vi "Vision Compression AE.vi"(7 "Update":bool, 10 "Quality (750)":i32=750) -> (2 "Quality out":i32, 5 "Compression":i32)   [LabVIEW 2023]
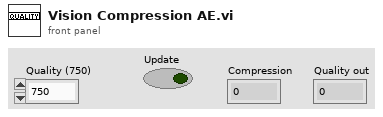
[diagram p1: front panel]
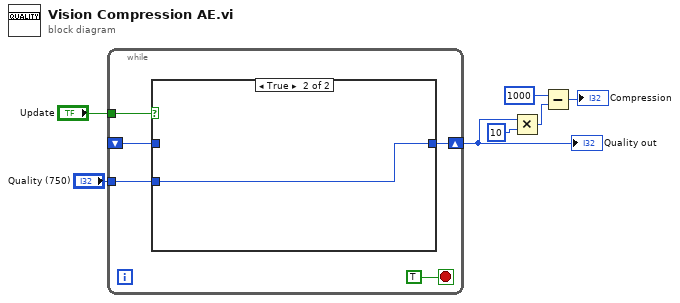
[diagram p0: block diagram]
diagram:
  n1 = while {
    shift-right: [w10] -> w4
    shift-left: _ -> [w9]
    tunnel: "Update" -> [w12]
    tunnel: "Quality (750)" -> [w11]
    stop <- TRUE stop-if-true
    n2 = case shown="True" w12 {
      tunnel: w11 -> [_ w14]
      tunnel: [w13 w14] -> w10
      tunnel: w9 -> [w13 _]
      frame False {
      }
      frame True {
      }
    }
  }
  "Quality out" <- w4
  n3 = Multiply(x=w4, y=10) -> (x*y=w2:i32)
  n4 = Subtract(x=1000 ("Quality (750)"), y=w2) -> (x-y=→"Compression":i32)
